vi "reconnect to command stream delayed message.vi"(8 "error in (no error)":errorcluster, 11 "RT Queues":T1={"RT Message"=refnum, "RT Comms"=refnum, "RT Data"=refnum, "RT FIFO"=refnum, "message scheduler"=refnum}) -> (3 "schedule ID":u32)   [LabVIEW 2018]
uses:
  Queue VIs/En-queue RT comms element.vi
  Chris VIs/Message Scheduler/message scheduler.lvclass
  Type Defs/Queues cluster.ctl
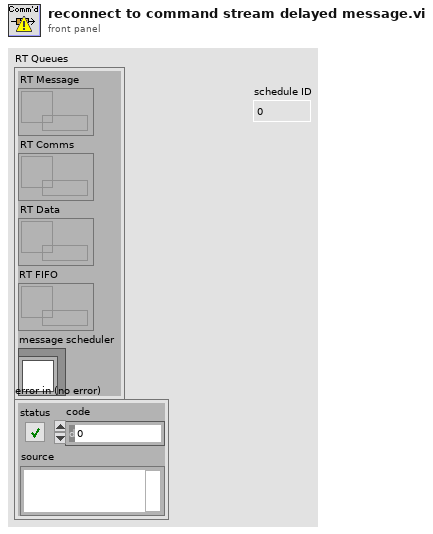
[diagram p1: front panel]
types:
  T1 = typedef "Queues cluster.ctl" = cluster{"RT Message":refnum<queue>, "RT Comms":refnum<queue>, "RT Data":refnum<queue>, "RT FIFO":refnum<queue>, "message scheduler":refnum<class "message scheduler.lvclass">}
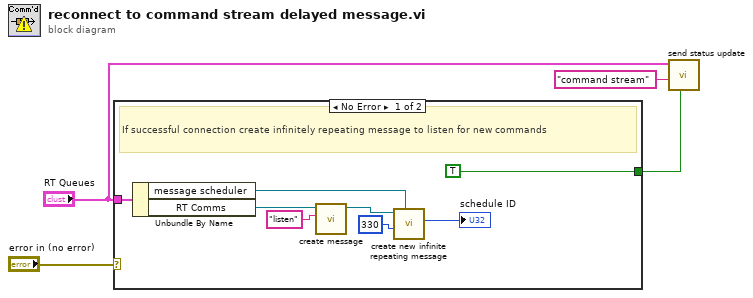
[diagram p0: block diagram]
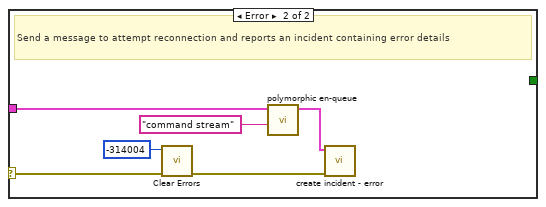
[diagram p2: hidden frame]
diagram:
  n1 = case shown="No Error" "error in (no error)" {
    selector: "error in (no error)" -> [_ w15]
    tunnel: "RT Queues" -> [w12 w18]
    tunnel: [TRUE _] -> w1
    frame No Error {
      # "If successful connection create infinitely repeating message to listen for new commands"
      n2 = Unbundle By Name(w12) -> ("message scheduler"=w6:refnum<class "message scheduler.lvclass">, "RT Comms"=w10:refnum<queue>)
      n3 = call "create message.vi"("message"="listen", "queue ref"=w10) -> ("standard message out"=w8:refnum<class "standard message.lvclass">)  [unwired: 8 in, 1 out]
      n4 = call "create new infinite repeating message.vi"("message scheduler"=w6, "ms delay"=u32 330, "message"=w8) -> ("schedule ID"=→"schedule ID":u32)  [unwired: 7 in, 1 out]
    }
    frame Error {
      # "Send a message to attempt reconnection and reports an incident containing error details"
      n5 = call <vilib>:"Clear Errors.vi"("error in (no error)"=w15, "specific error code to clear (0: all)"=-314004) -> ("error out"=w14:errorcluster)  [unwired: 4 in, 1 out]
      n6 = call-poly "polymorphic en-queue.vi"("Message"="command stream" ("message"), "RT Queues"=w18) -> ("RT Queues out"=w16:T1)  [unwired: 9 in]
      n7 = call "create incident - error.vi"("error"=w14, "RT Queues"=w16) -> ()  [unwired: 9 in, 1 out]
    }
  }
  n8 = call "send status update.vi"("status (F)"=w1, "subject"="command stream" ("Message"), "RT Queues"="RT Queues") -> ()  [unwired: 8 in, 1 out]
